vi "Get Node Path Type.vi"(8 "error in (no error)":errorcluster, 11 "Node ref in":refnum<k20>) -> (0 "error out":errorcluster, 1 "Found ?":bool, 2 "Path Type out":string, 3 "Node ref out":refnum<k20>)   [LabVIEW 2018, in ".LVLIBP CD XML Updater.lvlib" / "Project XML Editor.lvclass"]
uses:
  Project XML Editor.lvclass
  <vilib>/xml/Close Reference(Node).vi
  <vilib>/xml/NI_XML.lvlib
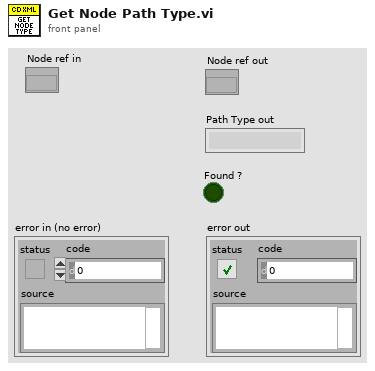
[diagram p1: front panel]
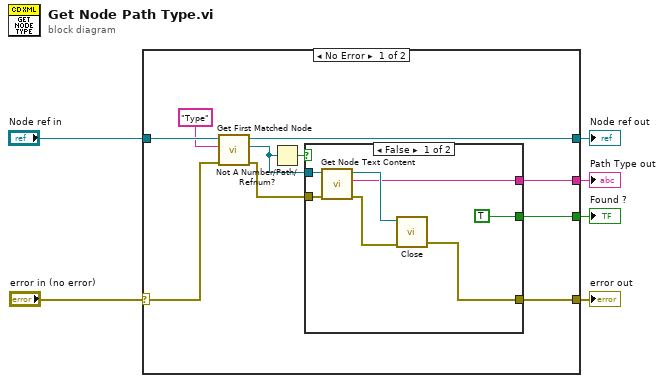
[diagram p0: block diagram]
diagram:
  n1 = case shown="No Error" "error in (no error)" {
    selector: "error in (no error)" -> [w12 w26]
    tunnel: "Node ref in" -> [w15 w25]
    tunnel: [w13 _] -> w5
    tunnel: [w11 w26] -> w3
    tunnel: [w10 w25] -> w2
    tunnel: [w7 _] -> w1
    frame No Error {
      n2 = call <vilib>:"Get First Matched Node.vi"("error in (no error)"=w12, "XPath expression"="Type", "node in"=w15) -> ("error out"=w16:errorcluster, "node result"=w9:refnum<k20>, "node out"=w10:refnum<k20>)  [unwired: 6 in]
      n3 = Not A Number/Path/Refnum?(number/path/refnum=w9) -> (NaN/Path/Refnum?=w8:bool)
      n4 = case shown="False" w8 {
        tunnel: w16 -> [w23 w24]
        tunnel: [w20 _] -> w13
        tunnel: [w19 w24] -> w11
        tunnel: w9 -> [w18 _]
        tunnel: [TRUE _] -> w7
        frame False {
          n5 = call <vilib>:"Get Node Text Content.vi"("error in (no error)"=w23, "node in"=w18) -> ("error out"=w21:errorcluster, "node text"=w20:string, "node out"=w22:refnum<k20>)  [unwired: 7 in]
          n6 = call-poly <vilib>:"Close.vi"("error in (no error)"=w21, "node"=w22) -> ("error out"=w19:errorcluster)  [unwired: 7 in]
        }
        frame True {
        }
      }
    }
    frame Error {
    }
  }
  "Path Type out" <- w5
  "error out" <- w3
  "Node ref out" <- w2
  "Found ?" <- w1
